vi "Stop.vi"(6 "Teller":refnum<class "Teller.lvclass">, 8 "Error in":errorcluster, 9 "Parent Stopped":bool, 10 "Safe Stop":bool=TRUE, 11 "Stop jettl Msg in":refnum<class "Stop jettl Msg.lvclass">) -> (0 "Error out":errorcluster, 3 "Stop jettl Msg out":refnum<class "Stop jettl Msg.lvclass">)   [LabVIEW 2020, in "jettl.lvlib" / "Stop jettl Msg.lvlib" / "Stop jettl Msg.lvclass"]
uses:
  Stop jettl Msg.lvclass
  Teller/Teller.lvclass
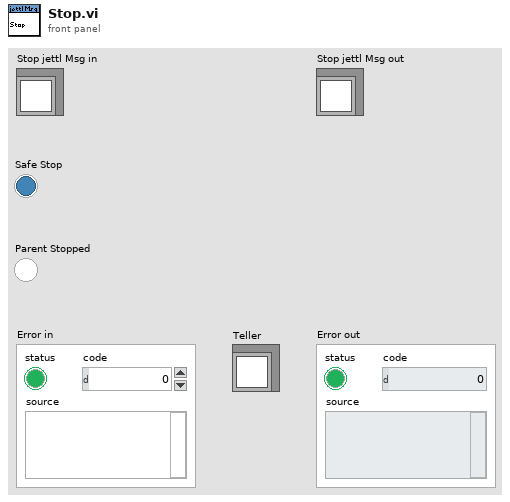
[diagram p1: front panel]
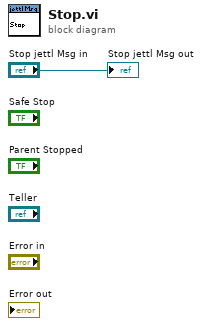
[diagram p0: block diagram]
diagram:
  "Stop jettl Msg out" <- "Stop jettl Msg in"
